vi "Command Loop - Apply Config.vi"(8 "error in":errorcluster, 10 "Data":u8[](array[numeric]), 11 "Queue Refs in":T1) -> (0 "error out":errorcluster, 2 "Response":string, 3 "Queue Refs out":T1)   [LabVIEW 2025, in "Runtime Configuration Support Example Engine.lvlib"]
uses:
  Runtime Configuration Support Example Engine.lvlib
  Shared/Compiled.Settings.ctl
  <vilib>/NI VeriStand/Custom Device API/Custom Device Item Ref.ctl
  <vilib>/NI VeriStand/Custom Device API/Custom Device API.lvlib
  Shared/Runtime Configuration Support Example Shared.lvlib
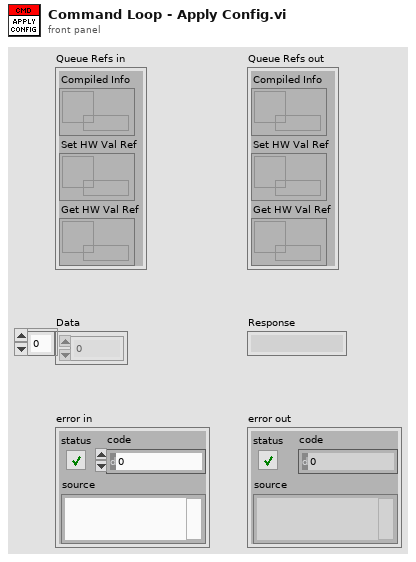
[diagram p1: front panel]
types:
  T1 = cluster{"Compiled Info":refnum<queue>, "Set HW Val Ref":refnum<queue>, "Get HW Val Ref":refnum<queue>}
  T2 = cluster{"Dynamic Config Status":bool, "Inports":i32[], "Outports":i32[], "Error":errorcluster}
  T3 = typedef "Runtime Configuration Support Example Shared.lvlib/Compiled.Settings.ctl" = cluster{"Name":string, "Inport SignalIDs":i32[], "Outport SignalIDs":i32[], "Inport Channel refs":T4[], "Outport Channel refs":T4[], "Inport Values":dbl[], "Outport Values":dbl[], "Device Error":errorcluster, "Dynamic Config Status":bool, "Response Ref":refnum<queue>}
  T4 = typedef "Custom Device API.lvlib/Custom Device Item Ref.ctl" = u64
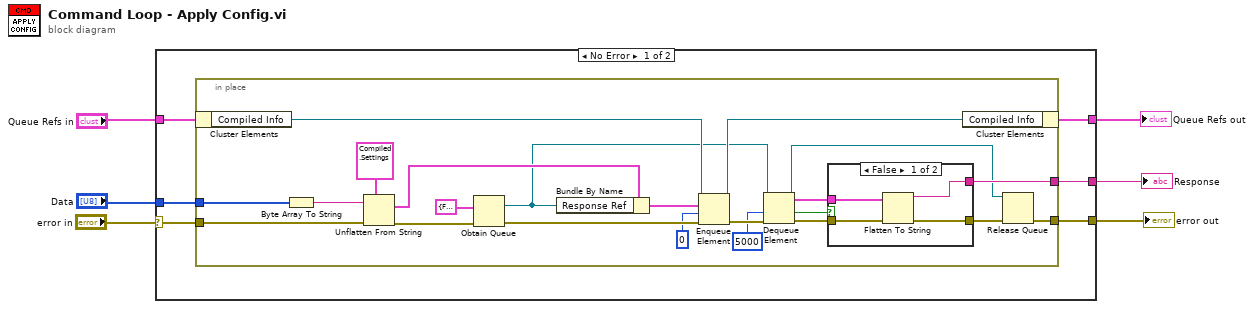
[diagram p0: block diagram]
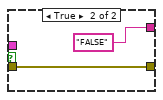
[diagram p2: hidden frame]
diagram:
  n1 = case shown="No Error" "error in" {
    selector: "error in" -> [w11 w42]
    tunnel: [w12 w42] -> w6
    tunnel: "Data" -> [w10 _]
    tunnel: [w9 _] -> w3
    tunnel: "Queue Refs in" -> [w8 w41]
    tunnel: [w7 w41] -> w1
    frame No Error {
      n2 = in-place {
        in-place-border: [w28] -> w12
        in-place-border: w11 -> [w31]
        in-place-border: w10 -> [w23]
        in-place-border: [w20] -> w9
        n3 = in-place-cluster #1(w8) -> ("Compiled Info"=w18:refnum<queue>)
        n4 = Byte Array To String(unsigned byte array=w23) -> (string=w24:string)
        n5 = Unflatten From String(type=T3 {"Name"="", "Inport SignalIDs"=[], "Outport SignalIDs"=[], "Inport Channel refs"=[], "Outport Channel refs"=[], "Inport Values"=[], "Outport Values"=[], "Device Error"={"status"=FALSE, "code"=0, "source"=""}, "Dynamic Config Status"=FALSE, "Response Ref"=refnum} ("Compiled.Settings"), binary string=w24, error in (no error)=w31) -> (value=w26:T3, error out=w34:errorcluster)  [unwired: 2 in, 1 out]
        n6 = Obtain Queue(element data type=T2 {"Dynamic Config Status"=FALSE, "Inports"=[], "Outports"=[], "Error"={"status"=FALSE, "code"=0, "source"=""}}, error in (no error)=w34) -> (queue out=w15:refnum<queue>, error out=w33:errorcluster)  [unwired: 3 in, 1 out]
        n7 = Bundle By Name(cluster=w26, "Response Ref"=w15) -> (w27:T3)
        n8 = Enqueue Element(queue=w18, element=w27, timeout in ms (-1)=0, error in (no error)=w33) -> (queue out=w17:refnum<queue>, error out=w30:errorcluster)  [unwired: 1 out]
        n9 = Dequeue Element(queue=w15, timeout in ms (-1)=5000, error in (no error)=w30) -> (queue out=w14:refnum<queue>, element=w22:T2, timed out?=w21:bool, error out=w32:errorcluster)
        n10 = case shown="False" w21 {
          tunnel: w22 -> [w35 _]
          tunnel: [w36 "FALSE"] -> w20
          tunnel: w32 -> [w38 w40]
          tunnel: [w37 w40] -> w29
          frame False {
            n11 = Flatten To String(anything=w35, error in (no error)=w38) -> (data string=w36:string, error out=w37:errorcluster)  [unwired: 2 in, 1 out]
          }
          frame True {
          }
        }
        n12 = in-place-cluster #1("Compiled Info"=w17) -> (w7:T1)
        n13 = Release Queue(queue=w14, error in (no error)=w29) -> (error out=w28:errorcluster)  [unwired: 1 in, 2 out]
      }
    }
    frame Error {
    }
  }
  "error out" <- w6
  "Response" <- w3
  "Queue Refs out" <- w1
